vi "Delacor_lib_QMH_Set Message Queue.vi"(8 "error in":errorcluster, 10 "Message Queue":refnum<queue>, 11 "Message Queue in":refnum<class "RQMHMessageQueue.lvclass">) -> (0 "error out":errorcluster, 3 "Message Queue out":refnum<class "RQMHMessageQueue.lvclass">)   [LabVIEW 2024, in "RQMHMessageQueue.lvclass"]
doc: "____\nDQMH Framework: Palette 7.1.0.1503\nCopyright (c) 2025, DQMH Consortium"
uses:
  RQMHMessageQueue.lvclass
  Delacor_lib_QMH_Message--cluster.ctl
  RQMHMessageQueue.lvclass/RQMHMessageQueue.ctl
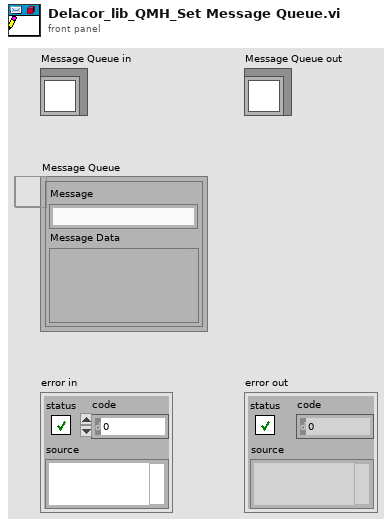
[diagram p1: front panel]
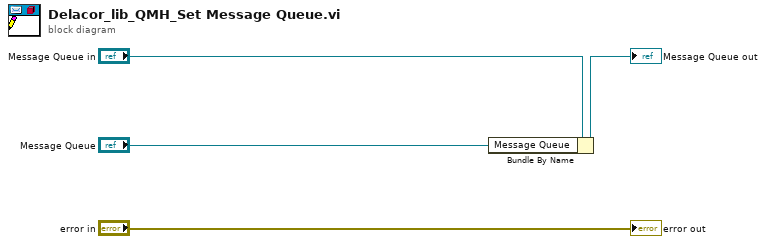
[diagram p0: block diagram]
diagram:
  n1 = Bundle By Name(cluster="Message Queue in", "Message Queue"="Message Queue") -> (→"Message Queue out":refnum<class "RQMHMessageQueue.lvclass">)
  "error out" <- "error in"
